vi "2D FFT Functional Global.vi"(6 "FFT Dimension":enum16{"1D FFT", "2D FFT"}(ring)=enum."2D FFT", 7 "FFT States":T2(ring), 8 "Error In":errorcluster, 9 "Real In":dbl[][][](array[numeric]), 10 "Dimension FFT":cluster{"Depth":u64, "Height":u64, "Width":u64}={"Depth"=1, "Height"=1000, "Width"=1024} {"Width" min=1; "Height" min=1; "Depth" min=1}, 11 "Device":T1) -> (0 "Error Out":errorcluster, 2 "Imag Data":dbl[][](array[numeric]), 3 "Real Data":dbl[][](array[numeric]), 4 "Labview Time":u32, 5 "OpenCLV Time":u32)   [LabVIEW 2012]
uses:
  Non-User VIs/Controls/Device ID.ctl
  FFT Global.ctl
  Non-User VIs/FFT/FFT Control.ctl
  Non-User VIs/FFT/FFT Types.ctl
  Non-User VIs/FFT/FFT Dimension.ctl
  Non-User VIs/Controls/Memory Object.ctl
  Non-User VIs/Controls/Memory ID.ctl
  User Controls/Array Dimensions.ctl
  Non-User VIs/Controls/Memory Type.ctl
  Non-User VIs/FFT/FFT Direction.ctl
  Non-User VIs/Write Memory/WriteMemory_64f.vi
  Non-User VIs/FFT/Compute FFT 64f.vi
  Non-User VIs/Read Memory/ReadMemory_64f.vi
  <vilib>/Analysis/2dsp.llb/2D Real FFT.vi
  <vilib>/Analysis/2dsp.llb/Real FFT.vi
  Non-User VIs/FFT/Delete FFT Plan 64f.vi
  Non-User VIs/Allocate Memory/AllocateMemory_64f.vi
  Non-User VIs/FFT/Create FFT Plan 64f.vi
  OpenCLV x64.lvlib
  <vilib>/Analysis/NI_AALPro.lvlib
panel:
  in  "FFT Dimension 2":enum16{"1D FFT", "2D FFT"}(ring)=enum."2D FFT"
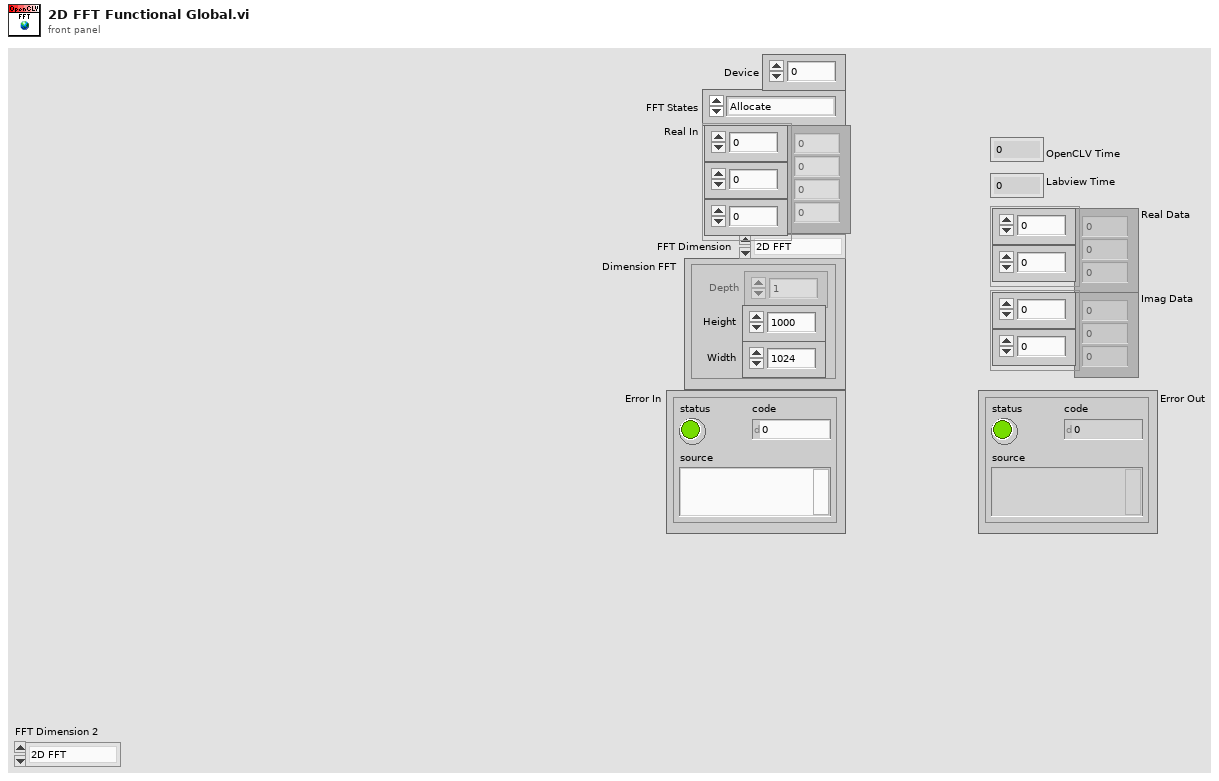
[diagram p1: front panel]
types:
  T1 = typedef "OpenCLV x64.lvlib/Device ID.ctl" = u64
  T2 = enum16{"Allocate", "Compute FFT and IFFT", "Compute Labivew FFT and IFFT", "Clean up"}
  T3 = typedef "FFT Global.ctl" = cluster{"FFT Object":T4, "IFFT Object":T4, "Memory Object":T7}
  T4 = typedef "OpenCLV x64.lvlib/FFT Control.ctl" = cluster{"Device ID":T1, "FFT Types":T5, "FFT Dim":T6, "Real":T7, "Imag":T7, "FFT Plan":u64, "FFT Direction":T11}
  T5 = typedef "OpenCLV x64.lvlib/FFT Types.ctl" = enum16{"Real to Hermitian", "Hermitian to Real", "Complex to Complex"}
  T6 = typedef "OpenCLV x64.lvlib/FFT Dimension.ctl" = enum16{"1D FFT", "2D FFT", "3D FFT"}
  T7 = typedef "OpenCLV x64.lvlib/Memory Object.ctl" = cluster{"Device ID":T1, "Memeroy ID":T8, "Dimension":T9, "Memory Type":T10}
  T8 = typedef "OpenCLV x64.lvlib/Memory ID.ctl" = u64
  T9 = typedef "Array Dimensions.ctl" = cluster{"Depth":u64, "Height":u64, "Width":u64}
  T10 = typedef "OpenCLV x64.lvlib/Memory Type.ctl" = enum16{"32f", "u8", "i8", "u16", "i16", "u32", "i32", "64f"}
  T11 = typedef "OpenCLV x64.lvlib/FFT Direction.ctl" = enum16{"Forward", "Reverse"}
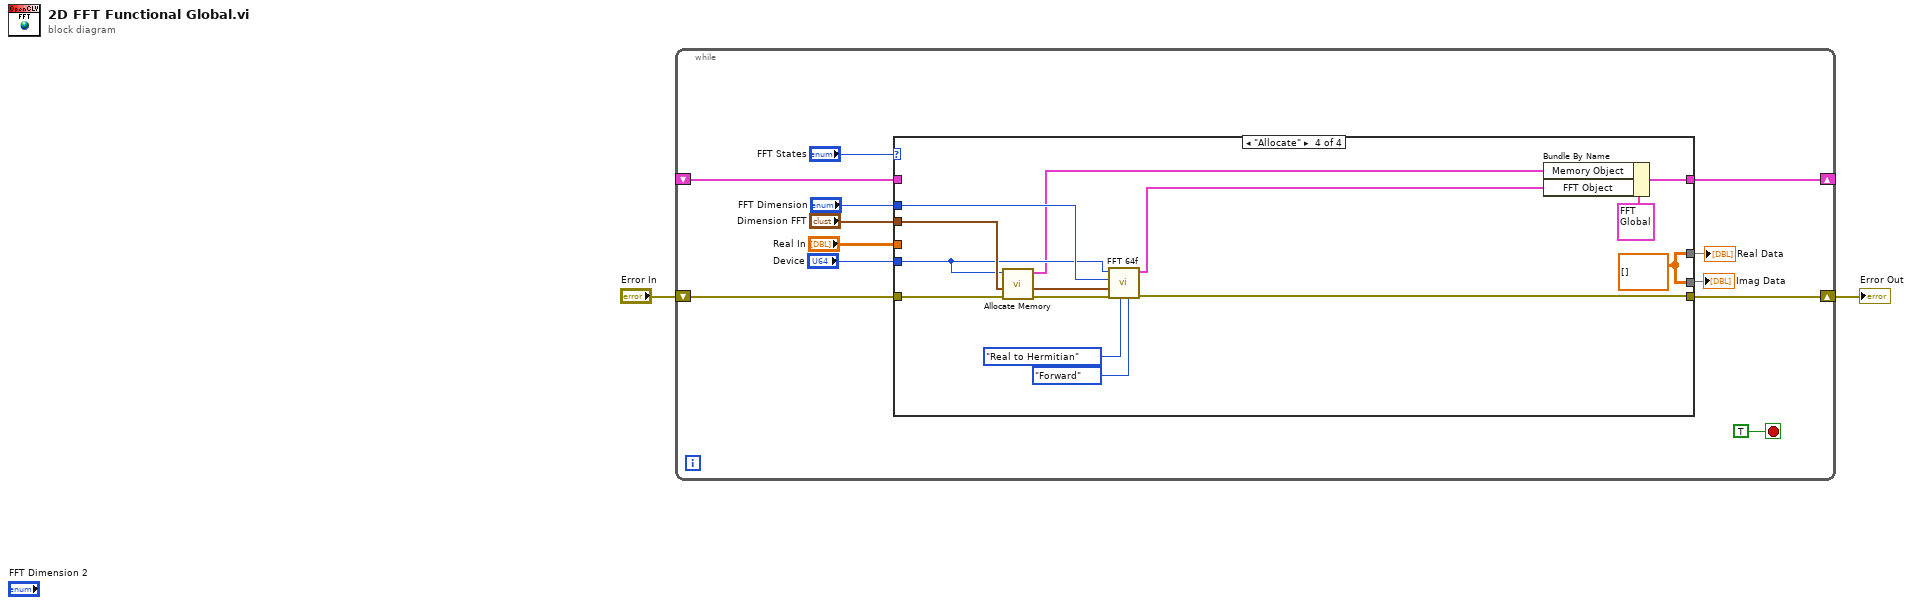
[diagram p0: block diagram]
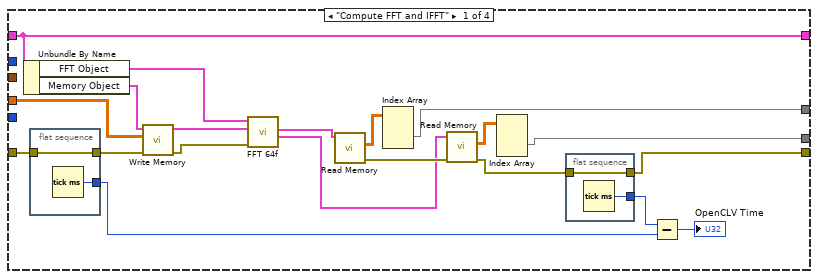
[diagram p2: hidden frame]
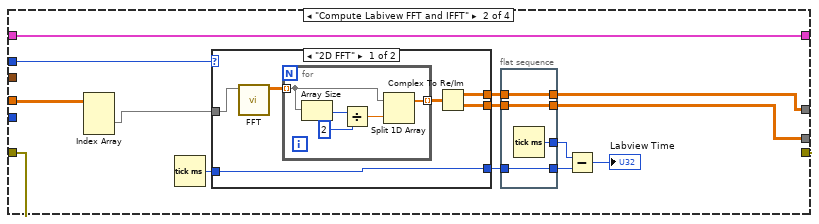
[diagram p3: hidden frame]
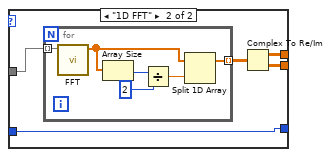
[diagram p4: hidden frame]
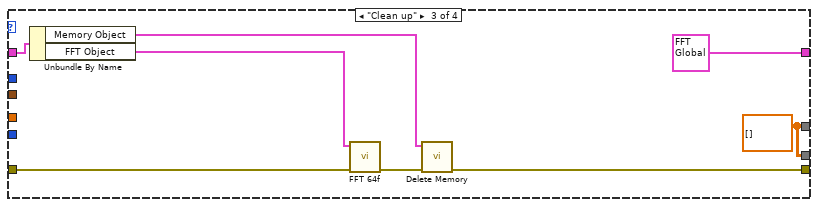
[diagram p5: hidden frame]
diagram:
  n1 = while {
    shift-right: [w8] -> w1
    shift-left: "Error In" -> [w9]
    shift-right: [w7] -> _
    shift-left: _ -> [w6]
    stop <- TRUE stop-if-true
    n2 = case shown="\"Allocate\"" "FFT States" {
      tunnel: "Dimension FFT" -> [_ _ _ w100]
      tunnel: "FFT Dimension" -> [_ w52 _ w92]
      tunnel: "Device" -> [_ _ _ w91]
      tunnel: w9 -> [w25 w49 w80 w99]
      tunnel: [w24 w49 w82 w88] -> w8
      tunnel: [w32 w43 T3 {"FFT Object"={"Device ID"=0, "FFT Types"=enum."Real to Hermitian", "FFT Dim"=enum."1D FFT", "Real"={"Device ID"=0, "Memeroy ID"=0, "Dimension"={"Depth"=0, "Height"=0, "Width"=0}, "Memory Type"=enum."32f"}, "Imag"={"Device ID"=0, "Memeroy ID"=0, "Dimension"={"Depth"=0, "Height"=0, "Width"=0}, "Memory Type"=enum."32f"}, "FFT Plan"=0, "FFT Direction"=enum."Forward"}, "IFFT Object"={"Device ID"=0, "FFT Types"=enum."Real to Hermitian", "FFT Dim"=enum."1D FFT", "Real"={"Device ID"=0, "Memeroy ID"=0, "Dimension"={"Depth"=0, "Height"=0, "Width"=0}, "Memory Type"=enum."32f"}, "Imag"={"Device ID"=0, "Memeroy ID"=0, "Dimension"={"Depth"=0, "Height"=0, "Width"=0}, "Memory Type"=enum."32f"}, "FFT Plan"=0, "FFT Direction"=enum."Forward"}, "Memory Object"={"Device ID"=0, "Memeroy ID"=0, "Dimension"={"Depth"=1, "Height"=1, "Width"=1}, "Memory Type"=enum."32f"}} ("Global Variable Locals") w98] -> w7
      tunnel: w6 -> [w32 w43 w86 _]
      tunnel: "Real In" -> [w34 w51 _ _]
      tunnel: [w18 w40 w79 w87] -> w3
      tunnel: [w17 w42 w79 w87] -> w4
      frame "Compute FFT and IFFT" {
        n3 = Unbundle By Name(w32) -> ("FFT Object"=w31:T4, "Memory Object"=w33:T7)
        n4 = flat-sequence {
          tunnel: [w36] -> w26
          tunnel: w25 -> [w36]
          tunnel: [w35] -> w23
          frame #0 {
            n5 = Tick Count (ms)() -> (millisecond timer value=w35:u32)
          }
        }
        n6 = call-poly "Write Memory.vi"("Error In"=w26, "Data In"=w34, "Memory Object In"=w33) -> ("Error Out"=w29:errorcluster, "Memory Object Out"=w30:T7)  [unwired: 6 in, 1 out]
        n7 = call-poly "FFT 64f.vi"("Error In"=w29, "Real In"=w30, "FFT Object"=w31) -> ("Imag Out"=w15:T7, "Real Out"=w16:T7)  [unwired: 4 in, 3 out]
        n8 = call-poly "Read Memory.vi"("Memory Object In"=w16) -> ("Error Out"=w20:errorcluster, "Data Out"=w27:dbl[][][])  [unwired: 7 in, 2 out]
        n9 = Index Array(array=w27) -> (element=w17:dbl[][])  [unwired: 3 in]
        n10 = call-poly "Read Memory.vi"("Error In"=w20, "Memory Object In"=w15) -> ("Error Out"=w19:errorcluster, "Data Out"=w21:dbl[][][])  [unwired: 6 in, 2 out]
        n11 = Index Array(array=w21) -> (element=w18:dbl[][])  [unwired: 3 in]
        n12 = flat-sequence {
          tunnel: [w37] -> w24
          tunnel: [w38] -> w28
          tunnel: w19 -> [w37]
          frame #0 {
            n13 = Tick Count (ms)() -> (millisecond timer value=w38:u32)
          }
        }
        n14 = Subtract(x=w28, y=w23) -> (x-y=→"OpenCLV Time":u32)
      }
      frame "Compute Labivew FFT and IFFT" {
        n15 = Index Array(array=w51) -> (element=w50:dbl[][])  [unwired: 3 in]
        n16 = Tick Count (ms)() -> (millisecond timer value=w48:u32)
        n17 = case shown="\"2D FFT\"" w52 {
          tunnel: w50 -> [w57 w70]
          tunnel: w48 -> [w62 w72]
          tunnel: [w62 w72] -> w47
          tunnel: [w59 w69] -> w41
          tunnel: [w58 w68] -> w39
          frame "2D FFT" {
            n18 = call-poly <vilib>:"FFT.vi"("X"=w57) -> ("FFT {X}"=w60:cdb[][])  [unwired: 9 in, 1 out]
            n19 = for {
              tunnel: w60 -> [w64] mode=indexing
              tunnel: [w63] -> w61 mode=indexing
              n20 = Array Size(array=w64) -> (size(s)=w67:i32)
              n21 = Divide(x=w67, y=2) -> (x/y=w65:dbl)
              n22 = Split 1D Array(array=w64, index=w65) -> (first subarray=w63:cdb[])  [unwired: 1 out]
            }
            n23 = Complex To Re/Im(x + iy=w61) -> (x=w59:dbl[][], y=w58:dbl[][])
          }
          frame "1D FFT" {
            n24 = for {
              tunnel: [w75] -> w71 mode=indexing
              tunnel: w70 -> [w74] mode=indexing
              n25 = call-poly <vilib>:"FFT.vi"("X"=w74) -> ("FFT {X}"=w73:cdb[])  [unwired: 9 in, 1 out]
              n26 = Array Size(array=w73) -> (size(s)=w78:i32)
              n27 = Divide(x=w78, y=2) -> (x/y=w76:dbl)
              n28 = Split 1D Array(array=w73, index=w76) -> (first subarray=w75:cdb[])  [unwired: 1 out]
            }
            n29 = Complex To Re/Im(x + iy=w71) -> (x=w69:dbl[][], y=w68:dbl[][])
          }
        }
        n30 = flat-sequence {
          tunnel: w47 -> [w56]
          tunnel: [w56] -> w46
          tunnel: [w55] -> w45
          tunnel: [w54] -> w42
          tunnel: w41 -> [w54]
          tunnel: [w53] -> w40
          tunnel: w39 -> [w53]
          frame #0 {
            n31 = Tick Count (ms)() -> (millisecond timer value=w55:u32)
          }
        }
        n32 = Subtract(x=w45, y=w46) -> (x-y=→"Labview Time":u32)
      }
      frame "Clean up" {
        w79 = dbl[][] [] ("Data Out")
        n33 = Unbundle By Name(w86) -> ("Memory Object"=w83:T7, "FFT Object"=w85:T4)
        n34 = call-poly "FFT 64f.vi"("Error In"=w80, "FFT Object"=w85) -> ("Error Out"=w84:errorcluster)  [unwired: 9 in]
        n35 = call "Delete Memory.vi"("Error In"=w84, "Memory Object In"=w83) -> ("Error Out"=w82:errorcluster)  [unwired: 8 in, 1 out]
      }
      frame "Allocate" {
        w87 = dbl[][] [] ("Data Out")
        n36 = call-poly "Allocate Memory.vi"("Error In"=w99, "Dimension"=w100, "Device In"=w91) -> ("Error Out"=w96:errorcluster, "Dimensions Out"=w95:T9, "Memory Object"=w90:T7)  [unwired: 6 in]
        n37 = call-poly "FFT 64f.vi"("Direction"=FFT_Direction."Forward", "FFT Types"=FFT_Types."Real to Hermitian", "Error In"=w96, "Dimension"=w95, "FFT Dimension"=w92, "Labview Device"=w91) -> ("Error Out"=w88:errorcluster, "FFT Object"=w89:T4)  [unwired: 3 in, 1 out]
        n38 = Bundle By Name(cluster=T3 {"FFT Object"={"Device ID"=0, "FFT Types"=enum."Real to Hermitian", "FFT Dim"=enum."1D FFT", "Real"={"Device ID"=0, "Memeroy ID"=0, "Dimension"={"Depth"=0, "Height"=0, "Width"=0}, "Memory Type"=enum."32f"}, "Imag"={"Device ID"=0, "Memeroy ID"=0, "Dimension"={"Depth"=0, "Height"=0, "Width"=0}, "Memory Type"=enum."32f"}, "FFT Plan"=0, "FFT Direction"=enum."Forward"}, "IFFT Object"={"Device ID"=0, "FFT Types"=enum."Real to Hermitian", "FFT Dim"=enum."1D FFT", "Real"={"Device ID"=0, "Memeroy ID"=0, "Dimension"={"Depth"=0, "Height"=0, "Width"=0}, "Memory Type"=enum."32f"}, "Imag"={"Device ID"=0, "Memeroy ID"=0, "Dimension"={"Depth"=0, "Height"=0, "Width"=0}, "Memory Type"=enum."32f"}, "FFT Plan"=0, "FFT Direction"=enum."Forward"}, "Memory Object"={"Device ID"=0, "Memeroy ID"=0, "Dimension"={"Depth"=1, "Height"=1, "Width"=1}, "Memory Type"=enum."32f"}} ("Global Variable Locals"), "Memory Object"=w90, "FFT Object"=w89) -> (w98:T3)
      }
    }
    "Real Data" <- w4
    "Imag Data" <- w3
  }
  "Error Out" <- w1
